vi "file_parsing.vi"(0 "File Path Control":path, 1 "line index":i32, 2 "error in":errorcluster) -> (3 "Waveform Chart":dbl(graph), 4 "String":string, 5 "index output":i32, 6 "error out":errorcluster)   [LabVIEW 2015]
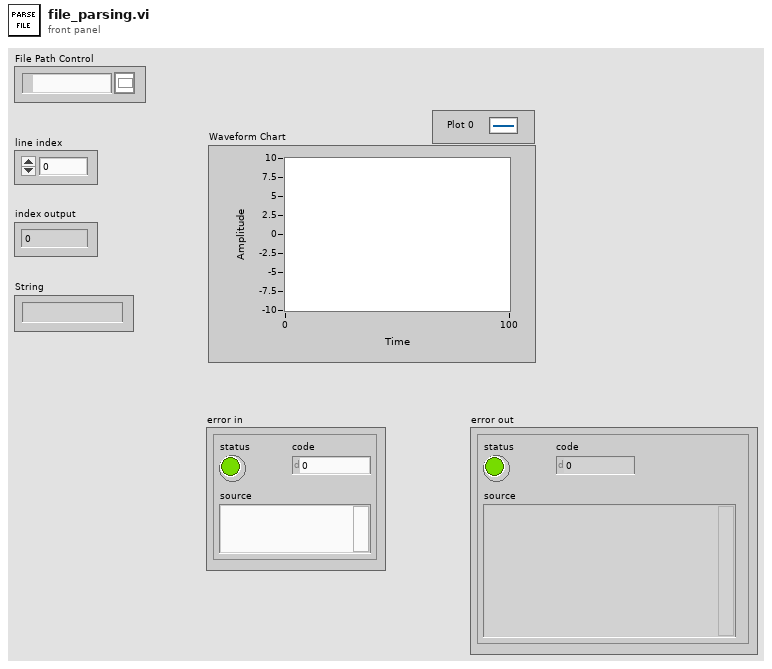
[diagram p1: front panel]
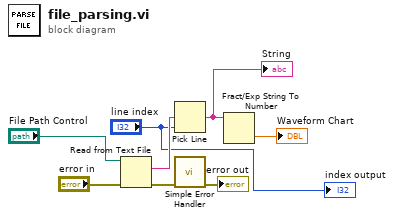
[diagram p0: block diagram]
diagram:
  n1 = Read from Text File(file (use dialog)="File Path Control", error in="error in") -> (text=w6:string, error out=w7:errorcluster)  [unwired: 2 in, 2 out]
  n2 = Pick Line(multi-line string=w6, line index="line index") -> (output string=w1:string)  [unwired: 1 in]
  "String" <- w1
  n3 = call <vilib>:"Simple Error Handler.vi"("error in (no error)"=w7) -> ("error out"=→"error out":errorcluster)  [unwired: 4 in, 4 out]
  n4 = Fract/Exp String To Number(string=w1) -> (number=→"Waveform Chart":dbl)  [unwired: 3 in, 1 out]
  "index output" <- "line index"
